vi "10-2 HP34401 n meas sol2.vi"(2 "Tc":sgl=1.0 format="%.2f", 3 "N":i32=5 min=1 max=500, 4 "Function (0:V DC)":u16(ring) items=["DC Voltage", "AC Voltage", "2--Wire Resistance", "4-Wire Resistance", "DC Current", "AC Current", "Frequency", "Period", "Continuity", "Diode Checking", "VDC: VDC Ratio"], 5 "GPIB address Multimeter":string="4") -> (0 "error out":errorcluster, 1 "Vet out":dbl[](array[numeric]) format="%.2f")   [LabVIEW 2012]
doc: "M. Ferrari M. Corti 2004\nMisura Ripetuta Vdc con HP34401A e DRV"
panel:
  # "MISURE RIPETUTE CON MULTIMETRO HP34401A ed USO dei VI del DRIVER di LabVIEW \n    Realizzare un VI che svolga le seguenti funzioni: \n   - configura il multimetro per una misura di tensione su un segnale sinusoidale in autoscala \n   - ripete la misura per un numero N (N=<100) di volte ad intervalli di tempo Tc, selezionabili da pannello\n   - memorizza i dati ottenuti in un vettore e segnala errori eventuali"
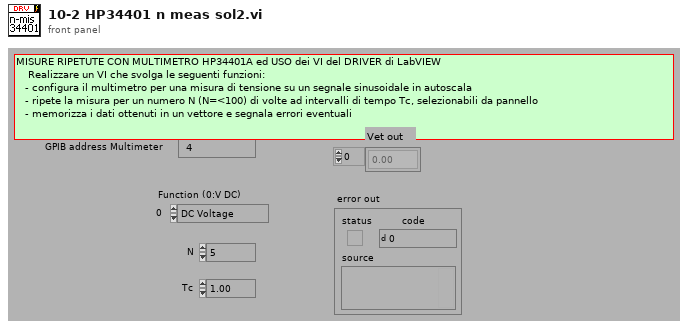
[diagram p1: front panel]
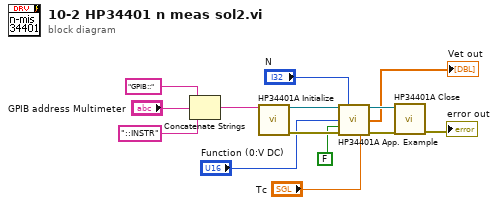
[diagram p0: block diagram]
diagram:
  n1 = Concatenate Strings("GPIB::", "GPIB address Multimeter", "::INSTR") -> (w11:string)
  n2 = call "HP34401A Initialize.vi"("Instr. Descriptor (GPIB::22)"=w11) -> ("VISA session"=w10:refnum<visa-resource-name>, "error out"=w9:errorcluster)  [unwired: 13 in]
  n3 = call "HP34401A App. Example.vi"("VISA session"=w10, "Samples (1)"="N", "Function (0:V DC)"="Function (0:V DC)", "Range/Resolution (T:Auto)"=FALSE, "error in (no error)"=w9, "Manual Delay (0)"="Tc") -> ("dup VISA session"=w7:refnum<visa-resource-name>, "Measurements"=→"Vet out":dbl[], "error out"=w6:errorcluster)  [unwired: 7 in]
  n4 = call "HP34401A Close.vi"("VISA session"=w7, "error in (no error)"=w6) -> ("error out"=→"error out":errorcluster)  [unwired: 13 in]
